vi "svm_get_libsvm_version.vi"(8 "error in (no error)":errorcluster) -> (0 "error out":errorcluster, 3 "version":i32)   [LabVIEW 2014]
uses:
  bin/x64/LVLibSVM.dll
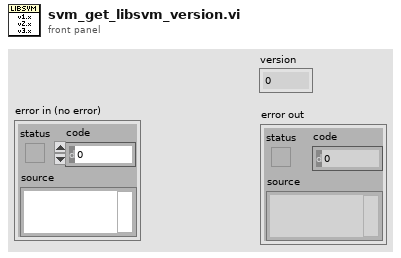
[diagram p1: front panel]
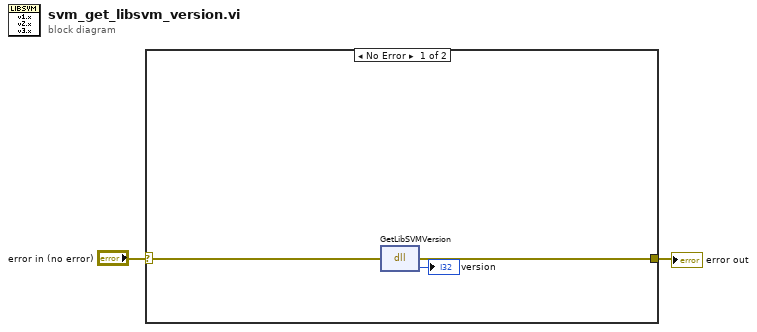
[diagram p0: block diagram]
diagram:
  n1 = case shown="No Error" "error in (no error)" {
    selector: "error in (no error)" -> [w5 w6]
    tunnel: [w4 w6] -> w2
    frame No Error {
      n2 = dll-call lib="C:/dev/LVLibSVM/LabVIEW/bin/x64/LVLibSVM.dll" fn="GetLibSVMVersion"(error in=w5) -> (error out=w4:errorcluster, "return type"=→"version":i32)  [unwired: 2 in, 1 out]
    }
    frame Error {
    }
  }
  "error out" <- w2
